vi "Replicate.vi"(8 "error in (no error)":errorcluster, 11 "Runner in":refnum<class "Runner.lvclass">) -> (0 "error out":errorcluster, 2 "New Type":refnum<class "Runner.lvclass">, 3 "Runner out":refnum<class "Runner.lvclass">, 5 "PlayerIdx":i32)   [LabVIEW 2014, in "Runner.lvclass"]
uses:
  Runner.lvclass
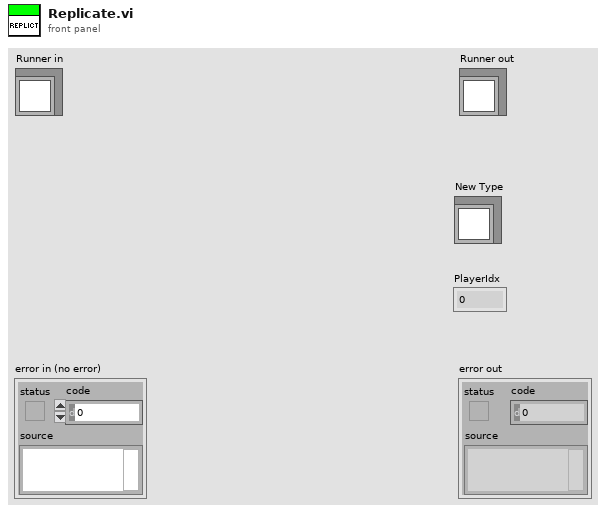
[diagram p1: front panel]
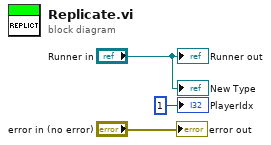
[diagram p0: block diagram]
diagram:
  "error out" <- "error in (no error)"
  "Runner out" <- "Runner in"
  "New Type" <- "Runner in"
  "PlayerIdx" <- 1 ("PlayerIdx")
